vi "RPLiDAR_축변환.vi"(8 "Theta(deg)":dbl[](array[numeric]), 11 "Distance(mm)":dbl[](array[numeric])) -> (0 "Y":dbl[](array[numeric]), 3 "X":dbl[](array[numeric]))   [LabVIEW 2024]
uses:
  <vilib>/Analysis/coordinate.llb/2D Cartesian Coordinate Rotation (Array).vi
  <vilib>/Analysis/NI_AALPro.lvlib
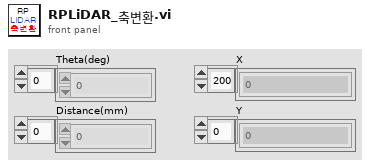
[diagram p1: front panel]
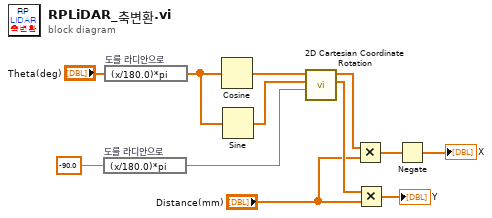
[diagram p0: block diagram]
diagram:
  n1 = expression code="(x/180.0)*pi" "도를 라디안으로"(-90.0 ("theta")) -> (w2:dbl)
  n2 = expression code="(x/180.0)*pi" "도를 라디안으로"("Theta(deg)") -> (w12:dbl[])
  n3 = Cosine(x=w12) -> (cos(x)=w11:dbl[])
  n4 = Sine(x=w12) -> (sin(x)=w10:dbl[])
  n5 = call-poly <vilib>:"2D Cartesian Coordinate Rotation.vi"("theta"=w2, "Y"=w10, "X"=w11) -> ("Y Out"=w7:dbl[], "X Out"=w8:dbl[])  [unwired: 6 in, 1 out]
  n6 = Multiply(x=w8, y="Distance(mm)") -> (x*y=w4:dbl[])
  n7 = Multiply(x=w7, y="Distance(mm)") -> (x*y=→"Y":dbl[])
  n8 = Negate(x=w4) -> (-x=→"X":dbl[])
